vi "Start Game.vi"(10 "Board Size":i32, 11 "MyTeam in":refnum<class "MyTeam.lvclass">) -> (3 "MyTeam out":refnum<class "MyTeam.lvclass">)   [LabVIEW 2020, in "The_Hill_Youth.lvlib" / "MyTeam.lvclass"]
uses:
  MyTeam.lvclass
  map_point.ctl
  MyTeam.lvclass/MyTeam.ctl
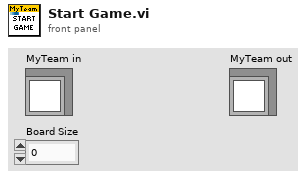
[diagram p1: front panel]
types:
  T1 = typedef "map_point.ctl" = cluster{"status":enum16{"unknown", "frind", "enemy", "empty"}, "plans":enum16{"stay", "duplicate", "attack", "move to", "no plans"}, "age":dbl}
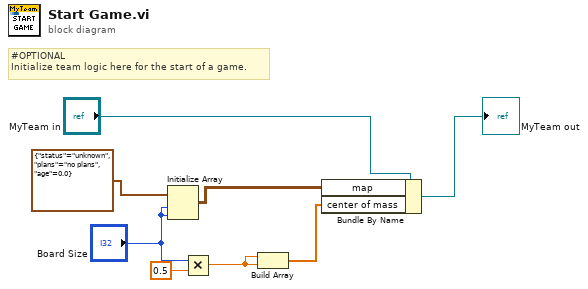
[diagram p0: block diagram]
diagram:
  # "#OPTIONAL\nInitialize team logic here for the start of a game."
  n1 = Initialize Array(T1 {"status"=enum."unknown", "plans"=enum."no plans", "age"=0.0} ("cluster"), "Board Size", "Board Size") -> (w5:T1[][])
  n2 = Multiply(x="Board Size", y=0.5) -> (x*y=w2:dbl)
  n3 = Build Array(w2, w2) -> (w1:dbl[])
  n4 = Bundle By Name(cluster="MyTeam in", "map"=w5, "center of mass"=w1) -> (→"MyTeam out":refnum<class "MyTeam.lvclass">)
